vi "Move.vi"(10 "Piece":i32[][](array[numeric]), 11 "Enum":enum16{"Up", "Left", "Right", "Down"}(ring)) -> (2 "New piece":i32[][](array[numeric]))   [LabVIEW 2014]
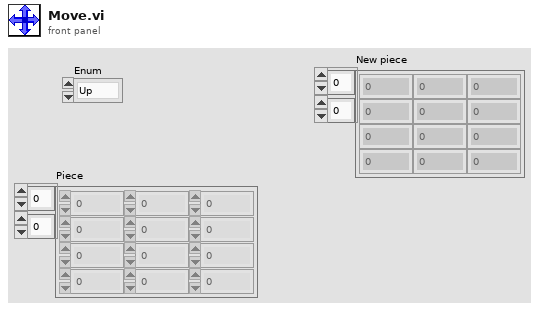
[diagram p1: front panel]
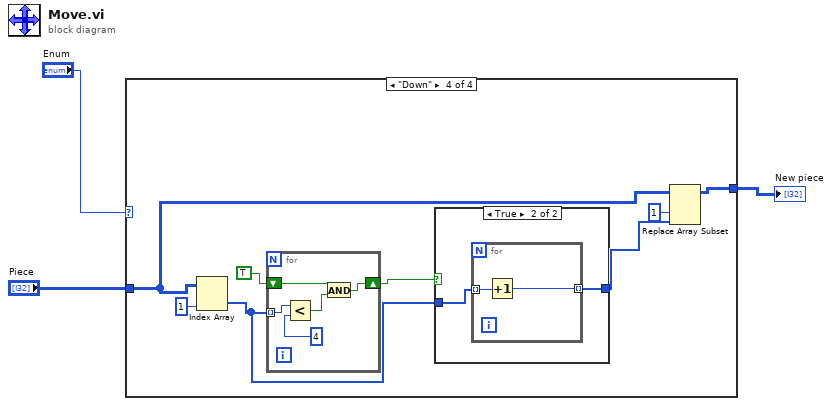
[diagram p0: block diagram]
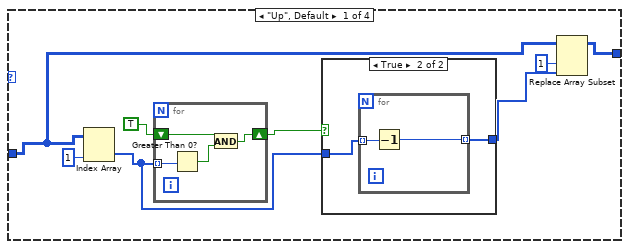
[diagram p2: hidden frame]
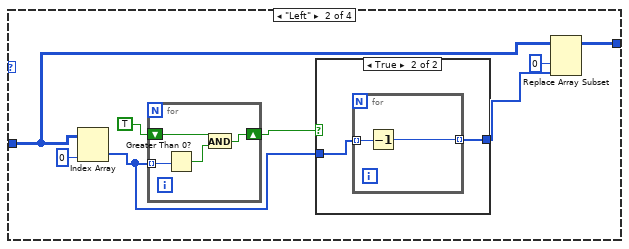
[diagram p4: hidden frame]
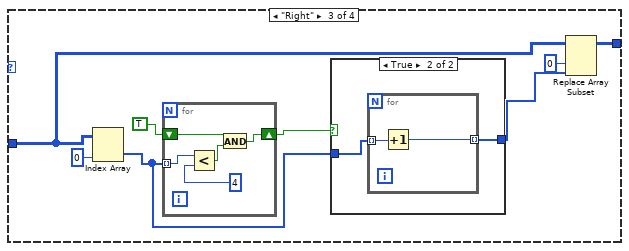
[diagram p6: hidden frame]
diagram:
  n1 = case shown="\"Down\"" "Enum" {
    tunnel: "Piece" -> [w5 w24 w39 w57]
    tunnel: [w4 w21 w38 w56] -> w1
    frame "Up", Default {
      n2 = Index Array(array=w5, index (col)=1 ("disabled index (col)")) -> (element=w9:i32[])  [unwired: 1 in]
      n3 = for {
        tunnel: w9 -> [w20] mode=indexing
        shift-right: [w19] -> w8
        shift-left: TRUE -> [w17]
        n4 = Greater Than 0?(x=w20) -> (x > 0?=w18:bool)
        n5 = And(x=w17, y=w18) -> (x .and. y?=w19:bool)
      }
      n6 = case shown="True" w8 {
        tunnel: w9 -> [w12 w14]
        tunnel: [w12 w13] -> w10
        frame False {
        }
        frame True {
          n7 = for {
            tunnel: w14 -> [w16] mode=indexing
            tunnel: [w15] -> w13 mode=indexing
            n8 = Decrement(x=w16) -> (x-1=w15:i32)
          }
        }
      }
      n9 = Replace Array Subset(array=w5, new element=w10, index (col)=1 ("disabled index (col)")) -> (w4:i32[][])  [unwired: 1 in]
    }
    frame "Left" {
      n10 = Index Array(array=w24, index (col)=0 ("disabled index (col)")) -> (element=w25:i32[])  [unwired: 1 in]
      n11 = for {
        tunnel: w25 -> [w37] mode=indexing
        shift-right: [w36] -> w26
        shift-left: TRUE -> [w34]
        n12 = Greater Than 0?(x=w37) -> (x > 0?=w35:bool)
        n13 = And(x=w34, y=w35) -> (x .and. y?=w36:bool)
      }
      n14 = case shown="True" w26 {
        tunnel: w25 -> [w29 w31]
        tunnel: [w29 w30] -> w23
        frame False {
        }
        frame True {
          n15 = for {
            tunnel: w31 -> [w33] mode=indexing
            tunnel: [w32] -> w30 mode=indexing
            n16 = Decrement(x=w33) -> (x-1=w32:i32)
          }
        }
      }
      n17 = Replace Array Subset(array=w24, new element=w23, index (col)=0 ("disabled index (col)")) -> (w21:i32[][])  [unwired: 1 in]
    }
    frame "Right" {
      n18 = Index Array(array=w39, index (col)=0 ("disabled index (col)")) -> (element=w42:i32[])  [unwired: 1 in]
      n19 = for {
        tunnel: w42 -> [w52] mode=indexing
        shift-right: [w55] -> w43
        shift-left: TRUE -> [w53]
        n20 = Less?(x=w52, y=4) -> (x < y?=w54:bool)
        n21 = And(x=w53, y=w54) -> (x .and. y?=w55:bool)
      }
      n22 = case shown="True" w43 {
        tunnel: w42 -> [w46 w48]
        tunnel: [w46 w47] -> w41
        frame False {
        }
        frame True {
          n23 = for {
            tunnel: w48 -> [w50] mode=indexing
            tunnel: [w49] -> w47 mode=indexing
            n24 = Increment(x=w50) -> (x+1=w49:i32)
          }
        }
      }
      n25 = Replace Array Subset(array=w39, new element=w41, index (col)=0 ("disabled index (col)")) -> (w38:i32[][])  [unwired: 1 in]
    }
    frame "Down" {
      n26 = Index Array(array=w57, index (col)=1 ("disabled index (col)")) -> (element=w61:i32[])  [unwired: 1 in]
      n27 = for {
        tunnel: w61 -> [w70] mode=indexing
        shift-right: [w73] -> w60
        shift-left: TRUE -> [w71]
        n28 = Less?(x=w70, y=4) -> (x < y?=w72:bool)
        n29 = And(x=w71, y=w72) -> (x .and. y?=w73:bool)
      }
      n30 = case shown="True" w60 {
        tunnel: w61 -> [w64 w66]
        tunnel: [w64 w65] -> w62
        frame False {
        }
        frame True {
          n31 = for {
            tunnel: w66 -> [w68] mode=indexing
            tunnel: [w67] -> w65 mode=indexing
            n32 = Increment(x=w68) -> (x+1=w67:i32)
          }
        }
      }
      n33 = Replace Array Subset(array=w57, new element=w62, index (col)=1 ("disabled index (col)")) -> (w56:i32[][])  [unwired: 1 in]
    }
  }
  "New piece" <- w1
